vi "Check and Generate Path to Octave Executable.vi"(8 "error in (no error)":errorcluster, 11 "octave executable file or directory with executable":path=path "C:/Octave/Octave-4.0.0/bin") -> (0 "error out":errorcluster, 3 "path to exe":path)   [LabVIEW 2013, in "GOLPI library.lvlib"]
doc: "Checks path provided by user if exists. If file, consider it as Octave executable. If directory, try to look for octave-cli.exe or octave.exe. Return path to Octave executable or generate an error."
uses:
  GOLPI library.lvlib
  Type Definitions/Custom Error Codes Enum Type Def.vi
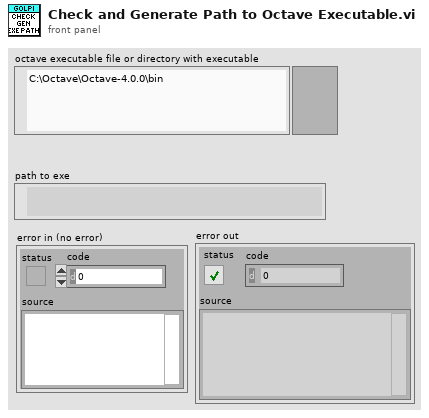
[diagram p1: front panel]
types:
  T1 = typedef "GOLPI library.lvlib/Custom Error Codes Enum Type Def.vi" = enum16{"no error", "00 working directory PAR1 missing", "01 octave binary PAR1 missing", "02 octave report error PAR1", "03 empty output last cmd PAR1", "04 missing temporary file PAR1", "05 pwd PAR 1 not exist", "10 var PAR1 not string, vect", "11 var PAR1 not num, scal, ~compl", "12 var PAR1 not num, scal, compl", "13 var PAR1 not num, vect, ~compl", "14 var PAR1 not num, vect, compl", "15 var PAR1 not num, mat, ~compl", "16 var PAR1 not num, mat, ~compl", "30 read timeout", "60 bitstream transport failed", "61 bitstream decode error PAR1", "62 bitstream cannot be set", "70 struct transfer not possible", "80 struct: cluster elem. PAR1 not implem.", "81 struct: structure field PAR1 not implem.", "82 struct: size mismatch of PAR1", "83 struct: type mismatch of PAR1", "98 internal error", "99 not finished"}
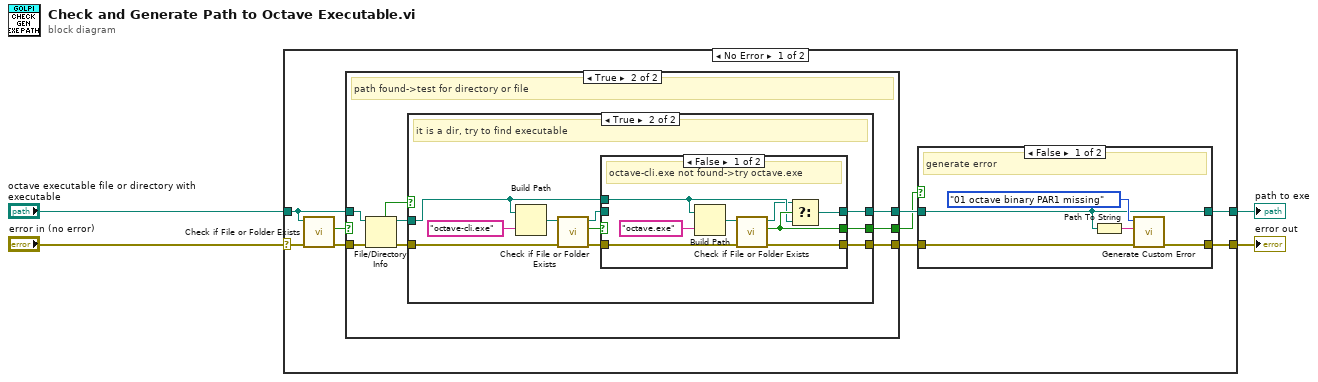
[diagram p0: block diagram]
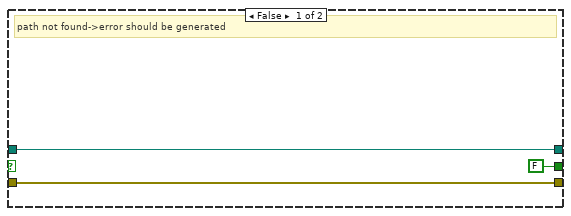
[diagram p3: hidden frame]
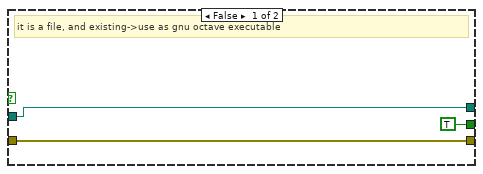
[diagram p4: hidden frame]
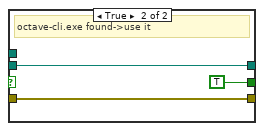
[diagram p5: hidden frame]
diagram:
  n1 = case shown="No Error" "error in (no error)" {
    selector: "error in (no error)" -> [w10 w57]
    tunnel: [w9 w57] -> w3
    tunnel: [w8 w56] -> w1
    tunnel: "octave executable file or directory with executable" -> [w6 w56]
    frame No Error {
      n2 = call <vilib>:"Check if File or Folder Exists.vi"("error in (no error)"=w10, "path"=w6) -> ("error out"=w13:errorcluster, "file or folder exists?"=w12:bool)  [unwired: 7 in, 1 out]
      n3 = case shown="True" w12 {
        tunnel: w6 -> [w23 w31]
        tunnel: w13 -> [w21 w30]
        tunnel: [w23 w28] -> w7
        tunnel: [FALSE w24] -> w5
        tunnel: [w21 w25] -> w11
        frame False {
          # "path not found->error should be generated"
        }
        frame True {
          # "path found->test for directory or file"
          n4 = File/Directory Info(path=w31, error in=w30) -> (path out=w27:path, directory=w29:bool, error out=w26:errorcluster)  [unwired: 4 out]
          n5 = case shown="True" w29 {
            tunnel: [w34 w35] -> w28
            tunnel: w27 -> [w34 w43]
            tunnel: w26 -> [w32 w39]
            tunnel: [w32 w37] -> w25
            tunnel: [TRUE w36] -> w24
            frame False {
              # "it is a file, and existing->use as gnu octave executable"
            }
            frame True {
              # "it is a dir, try to find executable"
              n6 = Build Path(base path=w43, name or relative path="octave-cli.exe" ("string")) -> (appended path=w42:path)
              n7 = call <vilib>:"Check if File or Folder Exists.vi"("error in (no error)"=w39, "path"=w42) -> ("error out"=w38:errorcluster, "file or folder exists?"=w41:bool, "dup path"=w40:path)  [unwired: 7 in]
              n8 = case shown="False" w41 {
                tunnel: w43 -> [w47 _]
                tunnel: w40 -> [_ w55]
                tunnel: [w46 w55] -> w35
                tunnel: w38 -> [w50 w54]
                tunnel: [w49 w54] -> w37
                tunnel: [w48 TRUE] -> w36
                frame False {
                  # "octave-cli.exe not found->try octave.exe"
                  n9 = Build Path(base path=w47, name or relative path="octave.exe" ("string")) -> (appended path=w51:path)
                  n10 = call <vilib>:"Check if File or Folder Exists.vi"("error in (no error)"=w50, "path"=w51) -> ("error out"=w49:errorcluster, "file or folder exists?"=w48:bool, "dup path"=w45:path)  [unwired: 7 in]
                  n11 = Select(t=w45, s=w48, f=w47) -> (s? t:f=w46:path)
                }
                frame True {
                  # "octave-cli.exe found->use it"
                }
              }
            }
          }
        }
      }
      n12 = case shown="False" w5 {
        tunnel: w11 -> [w18 w20]
        tunnel: [w17 w20] -> w9
        tunnel: [w15 w19] -> w8
        tunnel: w7 -> [w15 w19]
        frame False {
          # "generate error"
          n13 = Path To String(path=w15) -> (string=w14:string)
          n14 = call "Generate Custom Error.vi"("error in"=w18, "PAR1"=w14, "GOLPI error"=Custom_Error_Codes_Enum_Type_Def.vi."01 octave binary PAR1 missing") -> ("error out"=w17:errorcluster)  [unwired: 8 in]
        }
        frame True {
          # "some solution found, use it as Octave executable"
        }
      }
    }
    frame Error {
    }
  }
  "error out" <- w3
  "path to exe" <- w1
